vi "Take a Measurement.vi"(0 "Register Buses":refnum<class "ni579x Register Bus v1 Host.lvclass">[](array[class]), 11 "error in":errorcluster) -> (4 "Register Buses (out)":refnum<class "ni579x Register Bus v1 Host.lvclass">[](array[class]), 8 "measurement values":u16[](array[numeric]), 10 "measurement valid":bool, 15 "error out":errorcluster)   [LabVIEW 2012, in "ni579x Synchronization v1 Host.lvlib"]
uses:
  <instrlib>/ni579x/Synchronization/v1/Host/ni579x Synchronization v1 Host.lvlib
  <instrlib>/ni579x/Register Bus/v1/Host/ni579x Register Bus v1 Host.lvclass
  <instrlib>/ni579x/Synchronization/v1/Shared/ni579x Synchronization Register Addresses.ctl
  <instrlib>/ni579x/Register Bus/v1/Host/Public/Register Write.ctl
  <instrlib>/ni579x/Config/v1/Shared/Types/ni579x Register Bus Subsystem ID.ctl
  <instrlib>/ni579x/Register Bus/v1/Host/Public/Register Read Request.ctl
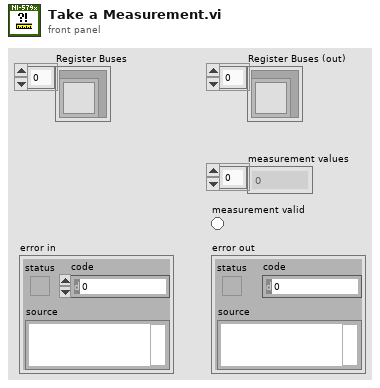
[diagram p1: front panel]
types:
  T1 = typedef "ni579x Register Bus Subsystem ID.ctl" = u8
  T2 = typedef "ni579x Synchronization Register Addresses.ctl" = enum16{"Signature", "Current Version", "Oldest Compatible Version", "Scratch Register", "sync.master", "sync.meas.enable", "sync.meas.ready", "sync.meas.arm", "sync.meas.valid", "sync.meas.value", "sync.cptr.adjust", "sync.cptr.period", "sync.meas.oversample factor"}
  T3 = typedef "ni579x Register Bus v1 Host.lvclass/Register Read Request.ctl" = cluster{"subsystem":u8, "address":u16}
  T4 = typedef "ni579x Register Bus v1 Host.lvclass/Register Write.ctl" = cluster{"subsystem":u8, "address":u16, "data":u32}
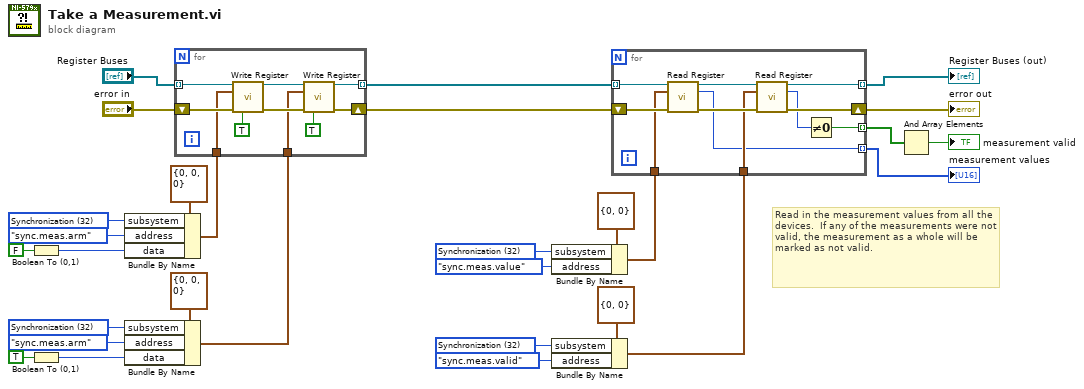
[diagram p0: block diagram]
diagram:
  w10 = T1 32 items=["FAM Register Operation"=0, "User Command"=16, "Synchronization"=32] ("Subsystem ID")
  w14 = T1 32 items=["FAM Register Operation"=0, "User Command"=16, "Synchronization"=32] ("Subsystem ID")
  w18 = T1 32 items=["FAM Register Operation"=0, "User Command"=16, "Synchronization"=32] ("Subsystem ID")
  w25 = T1 32 items=["FAM Register Operation"=0, "User Command"=16, "Synchronization"=32] ("Subsystem ID")
  # "Read in the measurement values from all the devices.  If any of the measurements were not valid, the measurement as a whole will be marked as not valid."
  n1 = Boolean To (0,1)(Boolean=FALSE ("sync.Master")) -> (0, 1=w27:i16)
  n2 = Boolean To (0,1)(Boolean=TRUE ("sync.Master")) -> (0, 1=w16:i16)
  n3 = Bundle By Name(cluster=T4 {"subsystem"=0, "address"=0, "data"=0} ("register write"), "subsystem"=w25, "address"=ni579x_Synchronization_Register_Addresses."sync.meas.arm" ("Synchronization Registers"), "data"=w27) -> (w28:T4)
  n4 = Bundle By Name(cluster=T4 {"subsystem"=0, "address"=0, "data"=0} ("register write"), "subsystem"=w18, "address"=ni579x_Synchronization_Register_Addresses."sync.meas.arm" ("Synchronization Registers"), "data"=w16) -> (w1:T4)
  n5 = for {
    tunnel: "Register Buses" -> [w39] mode=indexing
    tunnel: w28 -> [w37]
    tunnel: [w34] -> w12 mode=indexing
    shift-right: [w33] -> w21
    shift-left: "error in" -> [w38]
    tunnel: w1 -> [w31]
    n6 = call <instrlib>:"Write Register.vi"("session in"=w39, "register write"=w37, "error in"=w38, "wait until committed"=TRUE) -> ("session out"=w35:refnum<class "ni579x Register Bus v1 Host.lvclass">, "error out"=w32:errorcluster)  [unwired: 10 in]
    n7 = call <instrlib>:"Write Register.vi"("session in"=w35, "register write"=w31, "error in"=w32, "wait until committed"=TRUE) -> ("session out"=w34:refnum<class "ni579x Register Bus v1 Host.lvclass">, "error out"=w33:errorcluster)  [unwired: 10 in]
  }
  n8 = Bundle By Name(cluster=T3 {"subsystem"=0, "address"=0} ("register read request"), "subsystem"=w14, "address"=ni579x_Synchronization_Register_Addresses."sync.meas.value" ("Synchronization Registers")) -> (w8:T3)
  n9 = Bundle By Name(cluster=T3 {"subsystem"=0, "address"=0} ("register read request"), "subsystem"=w10, "address"=ni579x_Synchronization_Register_Addresses."sync.meas.valid" ("Synchronization Registers")) -> (w7:T3)
  n10 = for {
    tunnel: w12 -> [w48] mode=indexing
    tunnel: [w46] -> w2 mode=indexing
    shift-right: [w45] -> w3
    shift-left: w21 -> [w50]
    tunnel: w8 -> [w44]
    tunnel: w7 -> [w43]
    tunnel: [w41] -> w4 mode=indexing
    tunnel: [w40] -> w6 mode=indexing
    n11 = call <instrlib>:"Read Register.vi"("session in"=w48, "register read request"=w44, "error in"=w50) -> ("session out"=w47:refnum<class "ni579x Register Bus v1 Host.lvclass">, "data"=w41:u32, "error out"=w49:errorcluster)  [unwired: 10 in]
    n12 = call <instrlib>:"Read Register.vi"("session in"=w47, "register read request"=w43, "error in"=w49) -> ("session out"=w46:refnum<class "ni579x Register Bus v1 Host.lvclass">, "data"=w42:u32, "error out"=w45:errorcluster)  [unwired: 10 in]
    n13 = Not Equal To 0?(x=w42) -> (x != 0?=w40:bool)
  }
  "error out" <- w3
  "measurement values" <- w4
  "Register Buses (out)" <- w2
  n14 = And Array Elements(Boolean array=w6) -> (logical AND=→"measurement valid":bool)
